vi "Reference Signal Processing (Zero Crossing).vi"(7 "reset? (F)":bool, 8 "error in (no error)":errorcluster, 9 "filter for frequency measurement":T1={"enable filter? (T)"=TRUE, "passband edge frequency [Hz]"=55.0, "passband ripple [dB]"=0.1, "stopband edge frequency [Hz]"=85.0, "stopband attenuation [dB]"=60.0}, 10 "frequency range [Hz]":cluster{"minimum":dbl, "maximum":dbl}={"minimum"=45.0, "maximum"=55.0}, 11 "reference signal":waveform(dbl)={"t0"=timestamp(0 s since 1904-01-01), "dt"=2e-05, "Y"=[]}) -> (0 "error out":errorcluster, 2 "average frequency [Hz]":dbl, 3 "zero crossing information":T2, 4 "filtered reference signal":waveform(dbl)(graph)={"t0"=timestamp(-0.062370000000000037 s since 1904-01-01), "dt"=0.00044, "Y"=[]})   [LabVIEW 2013, in "NI_EP_Power Measurement.lvlib"]
doc: "Calculates the zero crossing times and the average fundamental frequency of a reference signal."
uses:
  <vilib>/addons/Electrical Power/Power Measurement/NI_EP_Power Measurement.lvlib
  <vilib>/addons/Electrical Power/Power Measurement/subVIs/ep_Filter Design.ctl
  <vilib>/addons/Electrical Power/PQ/Resampling/NI_EP_Resample_Host.lvlib
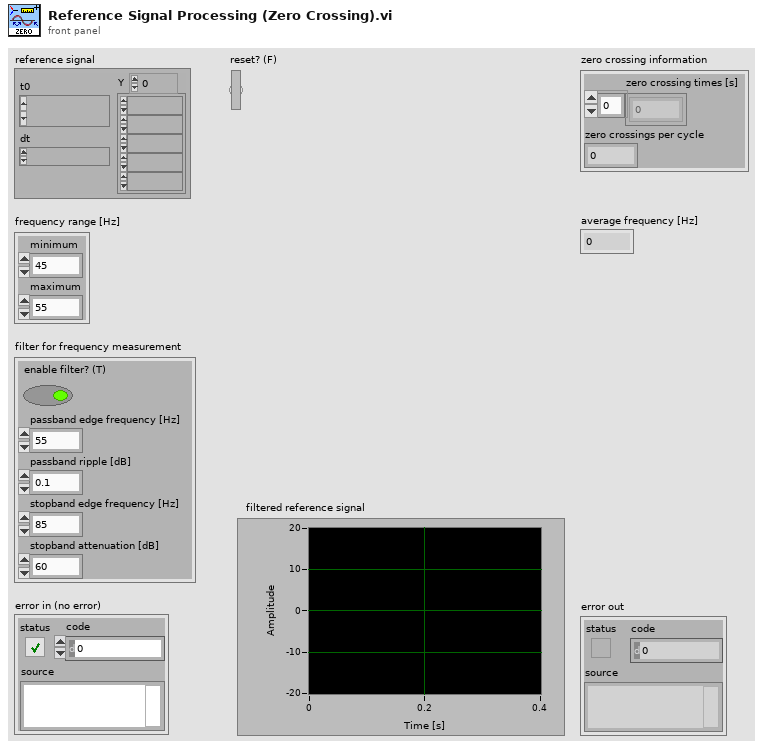
[diagram p1: front panel]
types:
  T1 = typedef "NI_EP_Power Measurement.lvlib/ep_Filter Design.ctl" = cluster{"enable filter? (T)":bool, "passband edge frequency [Hz]":dbl, "passband ripple [dB]":dbl, "stopband edge frequency [Hz]":dbl, "stopband attenuation [dB]":dbl}
  T2 = cluster{"zero crossing times [s]":dbl[], "zero crossings per cycle":u8}
  T3 = typedef "NI_EP_Resample_Host.lvlib/ep_Parameters.ctl" = cluster{"filter parameters":cluster{"enable filter":bool, "lp filter coefficients":dbl[], "bp filter coefficients":dbl[]}, "fs after decimation":dbl, "decimation factor":i32, "norminal frequency":dbl, "norminal hf prd samp":dbl, "lower hf prd samp":i32, "upper hf prd samp":i32}
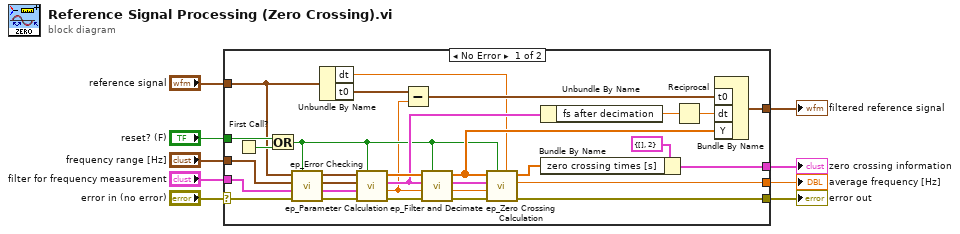
[diagram p0: block diagram]
diagram:
  n1 = case shown="No Error" "error in (no error)" {
    selector: "error in (no error)" -> [w36 w39]
    tunnel: "reset? (F)" -> [w37 _]
    tunnel: "filter for frequency measurement" -> [w35 _]
    tunnel: "frequency range [Hz]" -> [w34 _]
    tunnel: "reference signal" -> [w23 _]
    tunnel: [w25 _] -> w4
    tunnel: [w24 w39] -> w3
    tunnel: [w22 _] -> w2
    tunnel: [w19 _] -> w1
    frame No Error {
      n2 = First Call?() -> (First Call?: T/F=w38:bool)
      n3 = Or(x=w37, y=w38) -> (x .or. y?=w13:bool)
      n4 = call <vilib>:"ep_Error Checking.vi"("reset? (F)"=w13, "error in (no error)"=w36, "filter for frequency measurement"=w35, "frequency range [Hz]"=w34, "reference signal"=w23) -> ("error out"=w31:errorcluster, "dup filter for frequency measurement"=w30:T1, "dup frequency range [Hz]"=w32:cluster{"minimum":dbl, "maximum":dbl}, "dup reference signal"=w33:waveform(dbl))  [unwired: 3 in]
      n5 = Unbundle By Name(w23) -> ("dt"=w12:dbl, "t0"=w15:timestamp)
      n6 = call <vilib>:"ep_Parameter Calculation.vi"("reset? (F)"=w13, "error in (no error)"=w31, "filter for frequency measurement"=w30, "frequency range [Hz]"=w32, "reference signal"=w33) -> ("error out"=w28:errorcluster, "total group delay [s]"=w10:dbl, "parameters"=w18:T3, "data out"=w29:dbl[])  [unwired: 3 in]
      n7 = Subtract(x=w15, y=w10) -> (x-y=w14:timestamp)
      n8 = call <vilib>:"ep_Filter and Decimate.vi"("reset? (F)"=w13, "error in (no error)"=w28, "parameters"=w18, "data in"=w29) -> ("error out"=w27:errorcluster, "dup parameters"=w26:T3, "data out"=w20:dbl[])  [unwired: 5 in]
      n9 = call <vilib>:"ep_Zero Crossing Calculation.vi"("dt"=w12, "reset? (F)"=w13, "error in (no error)"=w27, "group delay"=w10, "parameters"=w26, "data in"=w20) -> ("error out"=w24:errorcluster, "average frequency [Hz]"=w25:dbl, "zero crossing positions [s]"=w11:dbl[])  [unwired: 3 in]
      n10 = Unbundle By Name(w18) -> ("fs after decimation"=w16:dbl)
      n11 = Bundle By Name(cluster=T2 {"zero crossing times [s]"=[], "zero crossings per cycle"=2} ("zero crossing information"), "zero crossing times [s]"=w11) -> (w22:T2)
      n12 = Reciprocal(x=w16) -> (1/x=w17:dbl)
      n13 = Bundle By Name("t0"=w14, "dt"=w17, "Y"=w20) -> (w19:waveform(dbl))  [unwired: 1 in]
    }
    frame Error {
    }
  }
  "error out" <- w3
  "zero crossing information" <- w2
  "average frequency [Hz]" <- w4
  "filtered reference signal" <- w1
